vi "读取表单内容.vi"(8 "错误输入（无错误）":errorcluster, 11 "选中区域引用输入":refnum<k7>) -> (0 "错误输出":errorcluster, 2 "数值":variant, 3 "引用输出":refnum<k7>)   [LabVIEW 2014, in "excel处理.lvlib"]
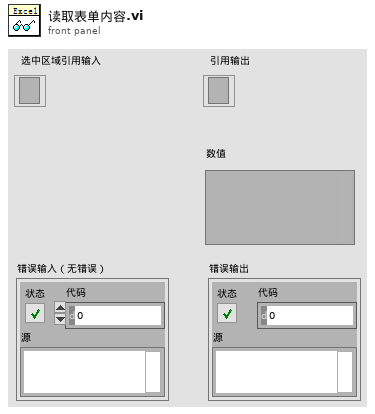
[diagram p1: front panel]
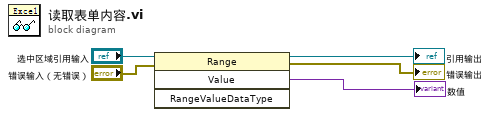
[diagram p0: block diagram]
diagram:
  n1 = invoke on="调用节点" class="Range" method="Value"(reference="选中区域引用输入", error in="错误输入（无错误）") -> (reference out=→"引用输出":refnum<k7>, error out=→"错误输出":errorcluster, "Value"=→"数值":variant)  [unwired: 2 in, 1 out]
